vi "public_device_occupy_server.vi"   [LabVIEW 2020]
uses:
  status/stop software.vi
  status/skip_latter.vi
  status/public_device_list.vi
  status/emergency stop.vi
  status/status of robot.vi
  status/status of pump.vi
  status/status of relay.vi
types:
  T1 = cluster{"ID":i32, "command":string, "skip command":string}
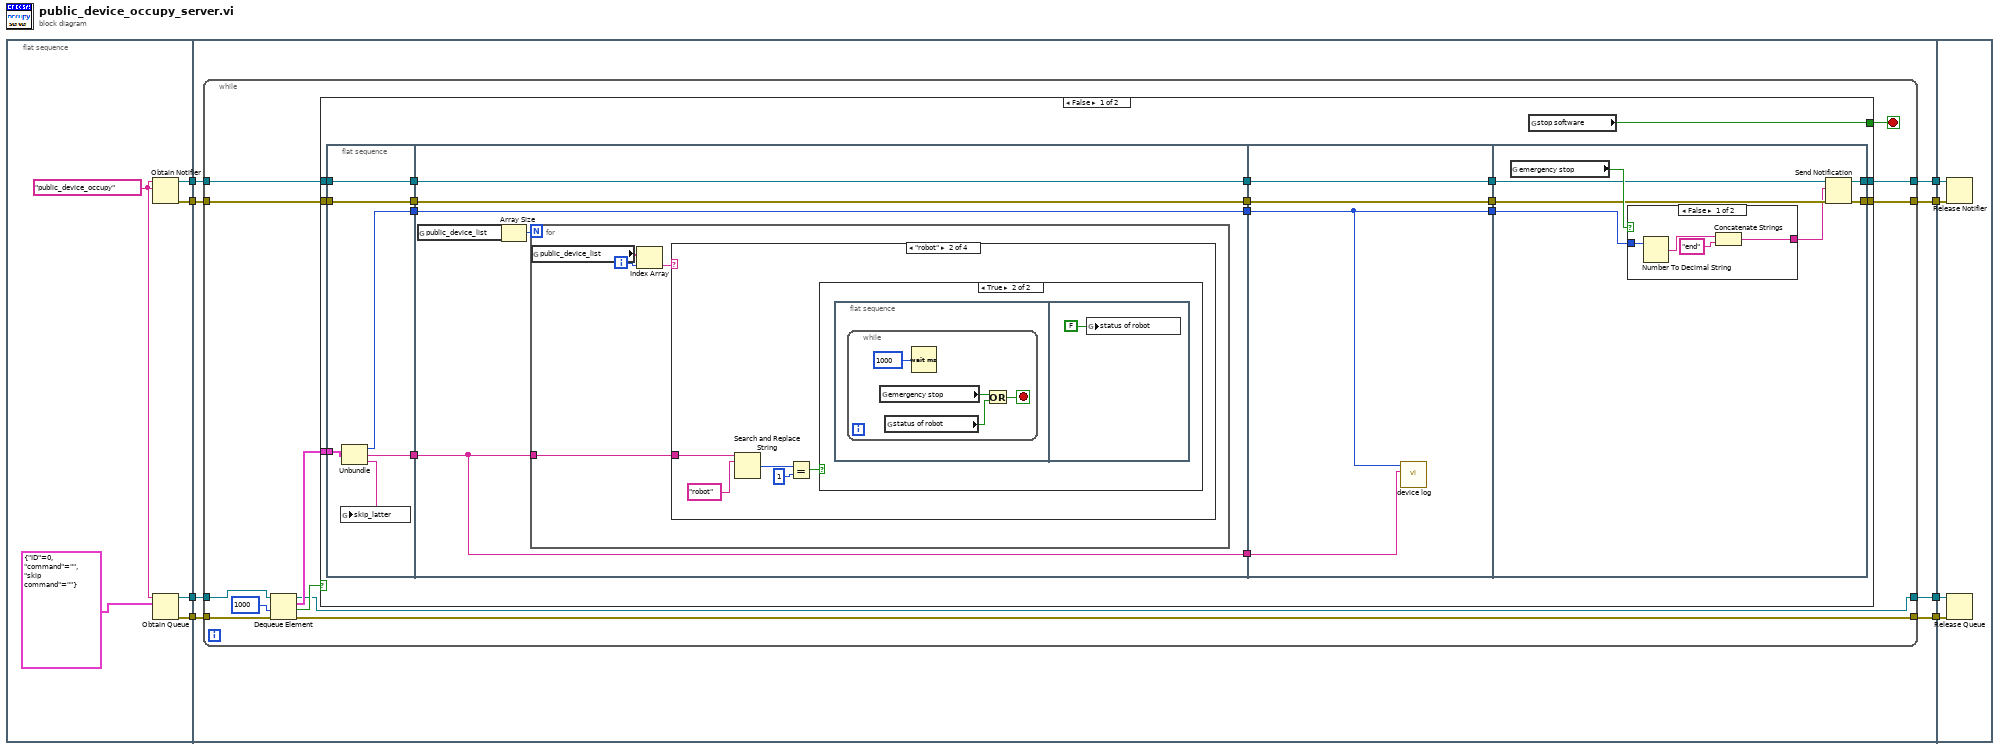
[diagram p0: block diagram]
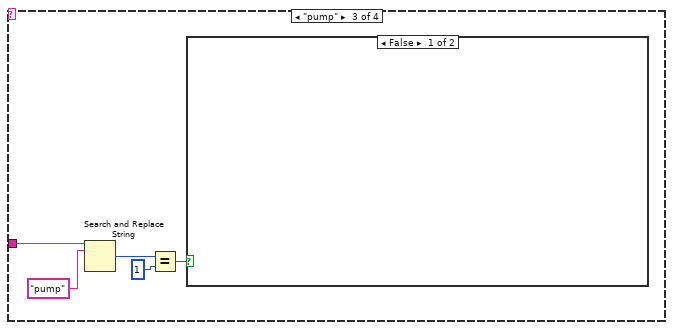
[diagram p4: hidden frame]
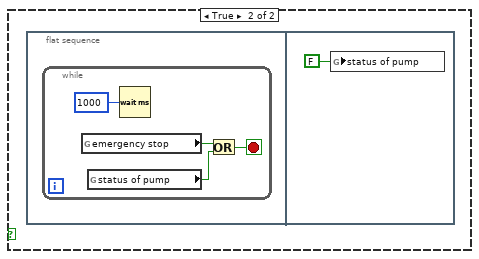
[diagram p5: hidden frame]
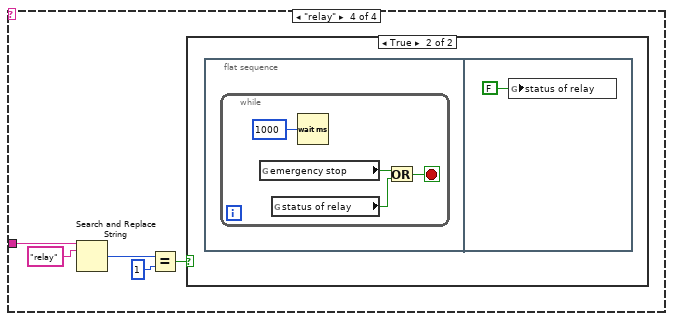
[diagram p6: hidden frame]
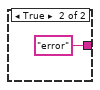
[diagram p8: hidden frame]
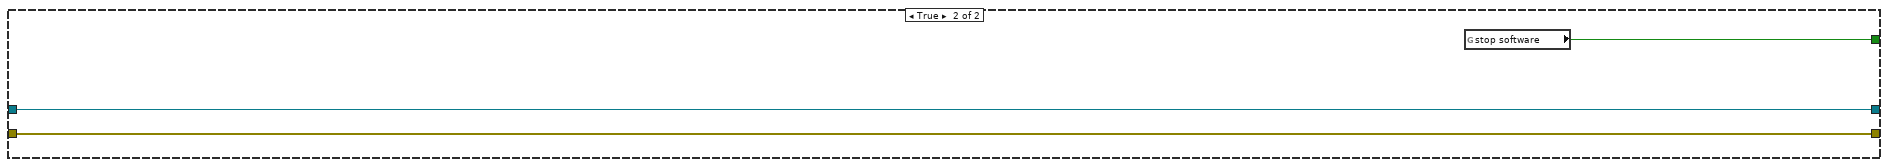
[diagram p9: hidden frame]
diagram:
  n1 = flat-sequence {
    tunnel: [w14] -> w8
    tunnel: [w13] -> w7
    tunnel: [w12] -> w6
    tunnel: [w10] -> w2
    tunnel: w8 -> [w22]
    tunnel: w7 -> [w21]
    tunnel: w6 -> [w20]
    tunnel: [w19] -> w5
    tunnel: [w18] -> w4
    tunnel: [w17] -> w3
    tunnel: w2 -> [w16]
    tunnel: [w15] -> w1
    tunnel: w5 -> [w120]
    tunnel: w4 -> [w119]
    tunnel: w3 -> [w118]
    tunnel: w1 -> [w117]
    frame #0 {
      w11 = "public_device_occupy" ("name (unnamed)")
      n2 = Obtain Notifier(name (unnamed)=w11, notification data type=w11) -> (notifier out=w12:refnum<notifier>, error out=w10:errorcluster)  [unwired: 2 in, 1 out]
      n3 = Obtain Queue(name (unnamed)=w11, element data type=T1 {"ID"=0, "command"="", "skip command"=""} ("参数")) -> (queue out=w14:refnum<queue>, error out=w13:errorcluster)  [unwired: 3 in, 1 out]
    }
    frame #1 {
      n4 = while {
        tunnel: w22 -> [w33]
        tunnel: w21 -> [w32]
        tunnel: w20 -> [w28]
        tunnel: [w27] -> w19
        tunnel: [w26] -> w18
        tunnel: [w25] -> w17
        tunnel: w16 -> [w24]
        tunnel: [w23] -> w15
        stop <- w30 stop-if-true
        n5 = Dequeue Element(queue=w33, timeout in ms (-1)=1000, error in (no error)=w32) -> (queue out=w26:refnum<queue>, element=w29:T1, timed out?=w31:bool, error out=w25:errorcluster)
        n6 = case shown="False" w31 {
          tunnel: [w51 w115] -> w30
          tunnel: w29 -> [w50 _]
          tunnel: w28 -> [w47 w116]
          tunnel: [w49 w116] -> w27
          tunnel: w24 -> [w46 w114]
          tunnel: [w44 w114] -> w23
          frame False {
            n7 = flat-sequence {
              tunnel: w50 -> [w57]
              tunnel: [w56] -> w48
              tunnel: w47 -> [w56]
              tunnel: w46 -> [w55]
              tunnel: [w55] -> w45
              tunnel: [w54] -> w43
              tunnel: [w53] -> w42
              tunnel: w48 -> [w63]
              tunnel: [w63] -> w41
              tunnel: w45 -> [w62]
              tunnel: [w62] -> w39
              tunnel: w43 -> [w61]
              tunnel: [w61] -> w37
              tunnel: w42 -> [w58]
              tunnel: [w58] -> w35
              tunnel: w41 -> [w101]
              tunnel: [w101] -> w40
              tunnel: w39 -> [w100]
              tunnel: [w100] -> w38
              tunnel: w37 -> [w99]
              tunnel: [w99] -> w36
              tunnel: w35 -> [w98]
              tunnel: [w107] -> w49
              tunnel: w40 -> [w106]
              tunnel: w38 -> [w105]
              tunnel: [w104] -> w44
              tunnel: w36 -> [w102]
              frame #0 {
                n8 = Unbundle(w57) -> ("ID"=w54:i32, "command"=w53:string, "skip command"=w52:string)
                n9 = global write "skip_latter.vi" "skip_latter"(w52) -> ()
              }
              frame #1 {
                n10 = global read "public_device_list.vi" "public_device_list"() -> (w60:string[])
                n11 = Array Size(array=w60) -> (size(s)=w59:i32)
                n12 = for {
                  N: w59 -> [_]
                  tunnel: w58 -> [w64]
                  i -> [w66]
                  n13 = global read "public_device_list.vi" "public_device_list"() -> (w67:string[])
                  n14 = Index Array(array=w67, index=w66) -> (element=w65:string)
                  n15 = case shown="\"robot\"" w65 {
                    tunnel: w64 -> [_ w68 w78 w89]
                    frame "False", Default {
                    }
                    frame "robot" {
                      n16 = Search and Replace String(input string=w68, search string="robot") -> (number of replacements=w72:i32)  [unwired: 6 in, 3 out]
                      n17 = Equal?(x=w72, y=1) -> (x = y?=w69:bool)
                      n18 = case shown="True" w69 {
                        frame False {
                        }
                        frame True {
                          n19 = flat-sequence {
                            frame #0 {
                              n20 = while {
                                stop <- w74 stop-if-true
                                n21 = global read "emergency stop.vi" "emergency stop"() -> (w75:bool)
                                n22 = global read "status of robot.vi" "status of robot"() -> (w73:bool)
                                n23 = Wait (ms)(milliseconds to wait=u32 1000) -> ()  [unwired: 1 out]
                                n24 = Or(x=w75, y=w73) -> (x .or. y?=w74:bool)
                              }
                            }
                            frame #1 {
                              n25 = global write "status of robot.vi" "status of robot"(FALSE ("status of robot")) -> ()
                            }
                          }
                        }
                      }
                    }
                    frame "pump" {
                      n26 = Search and Replace String(input string=w78, search string="pump") -> (number of replacements=w82:i32)  [unwired: 6 in, 3 out]
                      n27 = Equal?(x=w82, y=1) -> (x = y?=w79:bool)
                      n28 = case shown="False" w79 {
                        frame False {
                        }
                        frame True {
                          n29 = flat-sequence {
                            frame #0 {
                              n30 = while {
                                stop <- w84 stop-if-true
                                n31 = global read "emergency stop.vi" "emergency stop"() -> (w85:bool)
                                n32 = global read "status of pump.vi" "status of pump"() -> (w83:bool)
                                n33 = Wait (ms)(milliseconds to wait=u32 1000) -> ()  [unwired: 1 out]
                                n34 = Or(x=w85, y=w83) -> (x .or. y?=w84:bool)
                              }
                            }
                            frame #1 {
                              n35 = global write "status of pump.vi" "status of pump"(FALSE ("status of pump")) -> ()
                            }
                          }
                        }
                      }
                    }
                    frame "relay" {
                      n36 = Search and Replace String(input string=w89, search string="relay") -> (number of replacements=w92:i32)  [unwired: 6 in, 3 out]
                      n37 = Equal?(x=w92, y=1) -> (x = y?=w88:bool)
                      n38 = case shown="True" w88 {
                        frame False {
                        }
                        frame True {
                          n39 = flat-sequence {
                            frame #0 {
                              n40 = while {
                                stop <- w94 stop-if-true
                                n41 = global read "emergency stop.vi" "emergency stop"() -> (w95:bool)
                                n42 = global read "status of relay.vi" "status of relay"() -> (w93:bool)
                                n43 = Wait (ms)(milliseconds to wait=u32 1000) -> ()  [unwired: 1 out]
                                n44 = Or(x=w95, y=w93) -> (x .or. y?=w94:bool)
                              }
                            }
                            frame #1 {
                              n45 = global write "status of relay.vi" "status of relay"(FALSE ("status of relay")) -> ()
                            }
                          }
                        }
                      }
                    }
                  }
                }
              }
              frame #2 {
                n46 = call "device log.vi"("new element/subarray"=w98, "worker ID"=w99) -> ()  [unwired: 10 in]
              }
              frame #3 {
                n47 = global read "emergency stop.vi" "emergency stop"() -> (w108:bool)
                n48 = case shown="False" w108 {
                  tunnel: [w111 "error" ("notification")] -> w103
                  tunnel: w102 -> [w110 _]
                  frame False {
                    n49 = Number To Decimal String(number=w110) -> (decimal integer string=w109:string)  [unwired: 1 in]
                    n50 = Concatenate Strings(w109, "end" ("string")) -> (w111:string)
                  }
                  frame True {
                  }
                }
                n51 = Send Notification(notification=w103, notifier=w106, error in (no error)=w105) -> (notifier out=w107:refnum<notifier>, error out=w104:errorcluster)
              }
            }
            n52 = global read "stop software.vi" "stop software"() -> (w51:bool)
          }
          frame True {
            n53 = global read "stop software.vi" "stop software"() -> (w115:bool)
          }
        }
      }
    }
    frame #2 {
      n54 = Release Notifier(notifier=w120, error in (no error)=w117) -> ()  [unwired: 1 in, 3 out]
      n55 = Release Queue(queue=w119, error in (no error)=w118) -> ()  [unwired: 1 in, 3 out]
    }
  }
